vi "Serialize.vi"(8 "error in (no error)":errorcluster, 11 "Audit Event":refnum<class "Audit Event.lvclass">) -> (0 "error out":errorcluster, 3 "Serialized Audit Event":string)   [LabVIEW 2026, in "Audit Event.lvclass"]
uses:
  Audit Event.lvclass
  Audit Event.lvclass/Audit Event.ctl
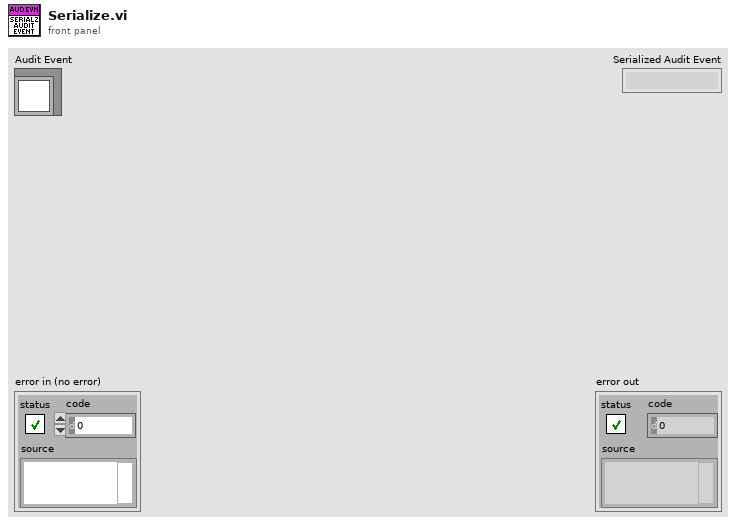
[diagram p1: front panel]
types:
  T1 = typedef "Audit Event Type Enum.ctl" = enum16{"Startup", "Shutdown", "Login", "Logout", "ReadinessCheck", "RunStarted", "RunFinished", "Error"}
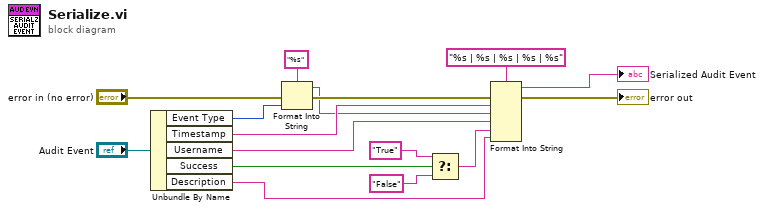
[diagram p0: block diagram]
diagram:
  n1 = Unbundle By Name("Audit Event") -> ("Event Type"=w14:T1, "Timestamp"=w10:string, "Username"=w8:string, "Success"=w7:bool, "Description"=w3:string)
  n2 = Format Into String(format string="%s", error in="error in (no error)", w14) -> (resulting string=w9:string, error out=w11:errorcluster)  [unwired: 1 in]
  n3 = Select(t="True", s=w7, f="False") -> (s? t:f=w4:string)
  n4 = Format Into String(format string="%s | %s | %s | %s | %s", error in=w11, w10, w9, w8, w4, w3) -> (resulting string=→"Serialized Audit Event":string, error out=→"error out":errorcluster)  [unwired: 1 in]
